vi "Persistent Data Menu.vi"() -> ()   [LabVIEW 2013]
panel:
  in  "File Name Prefix":string
  in  "Save Directory":path
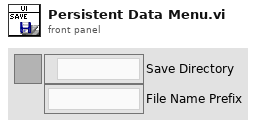
[diagram p1: front panel]
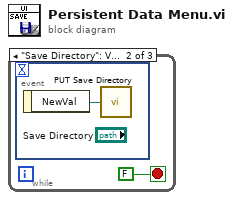
[diagram p0: block diagram]
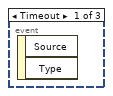
[diagram p2: hidden frame]
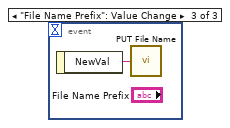
[diagram p3: hidden frame]
diagram:
  n1 = while {
    stop <- FALSE stop-if-true
    n2 = event shown="[1] \"Save Directory\": Value Change" {
      selector: _ -> [_ _ _]
      dyn-events: _ -> [_ _ _]
      timeout: _ -> [_ _ _]
      event Timeout {
        n3 = event-data() -> ()  [unwired: 1 in, 2 out]
      }
      event "Save Directory": Value Change {
        n4 = event-data() -> ("NewVal"=w2:path)  [unwired: 1 in]
        n5 = call "PUT Save Directory.vi"("Save Directory"=w2) -> ()
      }
      event "File Name Prefix": Value Change {
        n6 = event-data() -> ("NewVal"=w3:string)  [unwired: 1 in]
        n7 = call "PUT File Name.vi"("File Name"=w3) -> ()
      }
    }
  }
